vi "Get Wheel Type.vi"(8 "error in (no error)":errorcluster, 11 "mecanum wheel in":refnum<class "NI_Robotics_Mecanum Wheel.lvclass">) -> (0 "error out":errorcluster, 2 "wheel type":string, 3 "mecanum wheel out":refnum<class "NI_Robotics_Mecanum Wheel.lvclass">)   [LabVIEW 2017, in "NI_Robotics_Mecanum Wheel.lvclass"]
uses:
  <vilib>/robotics/Steering/Mecanum Wheel/NI_Robotics_Mecanum Wheel.lvclass
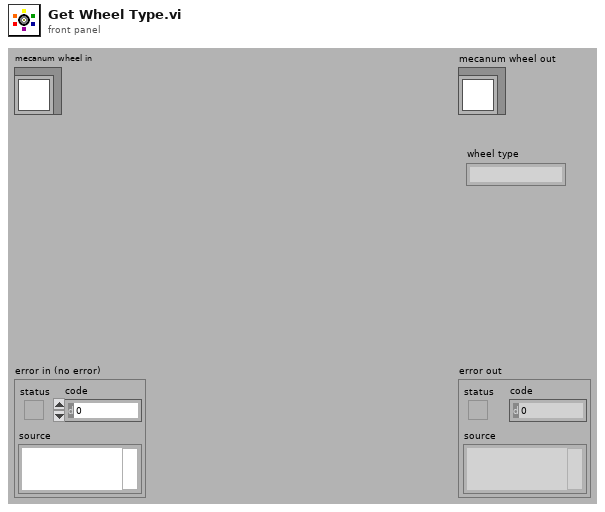
[diagram p1: front panel]
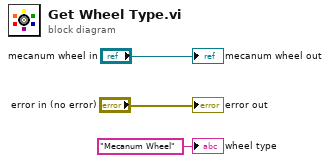
[diagram p0: block diagram]
diagram:
  "error out" <- "error in (no error)"
  "mecanum wheel out" <- "mecanum wheel in"
  "wheel type" <- "Mecanum Wheel" ("Wheel Type")
